vi "Initialise Waypoint GMap.vi"(7 "Aircraft ID":u8, 8 "error in (no error)":errorcluster, 11 "Main Map":refnum<k24>(container)) -> (0 "Error Out":errorcluster, 2 "Main Map Control Ref":refnum<k24>, 3 "Main map DLL Ref":refnum<k24>)   [LabVIEW 2014]
uses:
  C:/Robotic Systems/Products/AgFalcon/Software/Ground Station/Data/Mapping DLL/GMap.NET.WindowsForms.dll
  Data/Mapping DLL/GMap.NET.WindowsForms.dll
  C:/Robotic Systems/Products/AgFalcon/Software/Ground Station/Data/Mapping DLL/GMap.NET.Core.dll
  Data/Mapping DLL/GMap.NET.Core.dll
  Aircraft Information/Sub VI/Get Aircraft GPS.vi
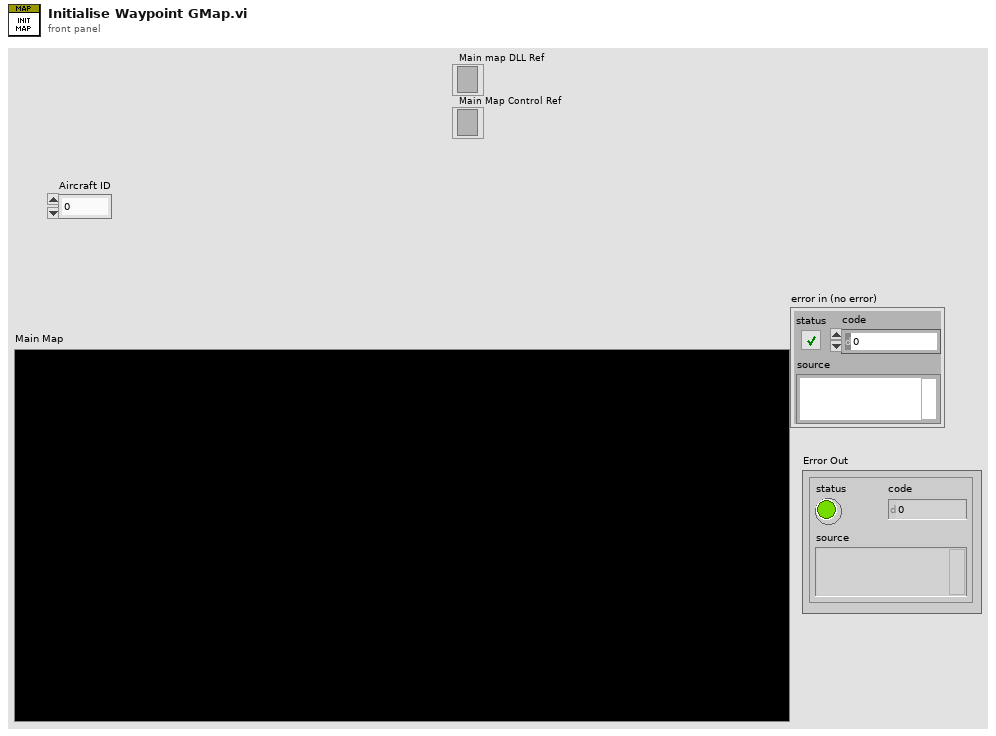
[diagram p1: front panel]
types:
  T1 = typedef "Aircraft GPS Data.ctl" = cluster{"Latitude (degrees)":dbl, "Longitude (degrees)":dbl, "Altitude (m)":dbl, "Fix Type":u8, "HDOP (cm)":u16, "VDOP (cm)":u16, "Ground Speed (m/s)":dbl, "Coarse Over Ground (degrees)":u16, "Number of Satellites":u8}
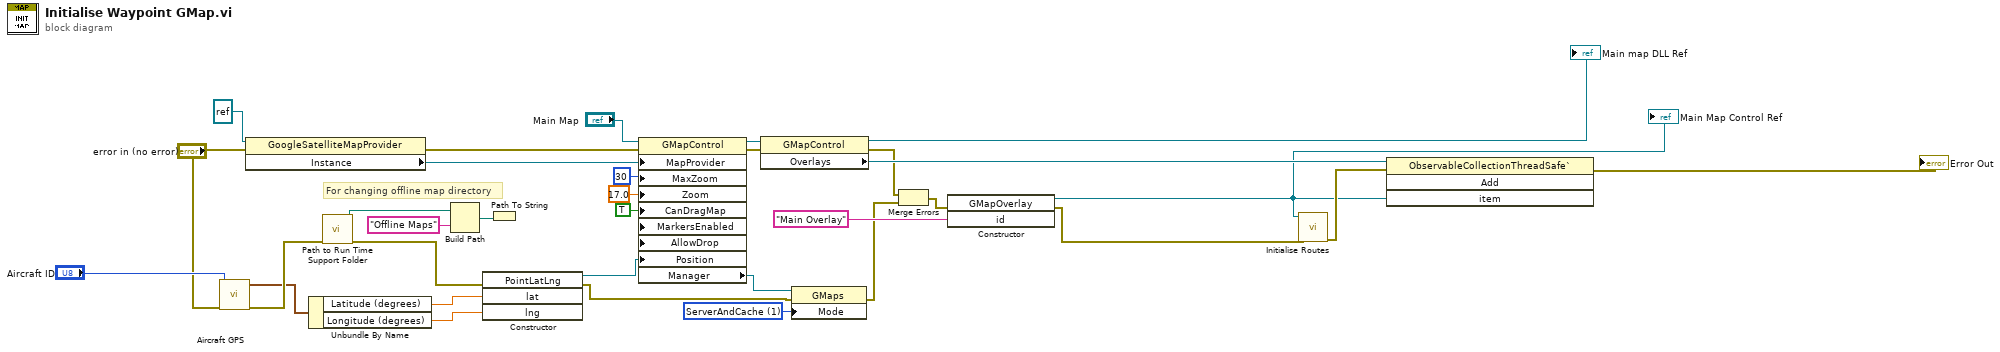
[diagram p0: block diagram]
diagram:
  w22 = 1 items=["ServerOnly", "ServerAndCache", "CacheOnly"] ("Mode")
  w27 = TRUE ("CanDragMap")
  # "For changing offline map directory"
  n1 = call-poly "Aircraft GPS.vi"("Error In"="error in (no error)", "Aircraft ID"="Aircraft ID") -> ("Error Out"=w4:errorcluster, "Aircraft GPS Data Out"=w3:T1)  [unwired: 8 in]
  n2 = property class="GoogleSatelliteMapProvider"(reference=refnum<k24> refnum (".NET Container Reference"), error in="error in (no error)") -> (error out=w33:errorcluster, "Instance"=w32:refnum<k24>)  [unwired: 1 out]
  n3 = Unbundle By Name(w3) -> ("Latitude (degrees)"=w2:dbl, "Longitude (degrees)"=w1:dbl)
  n4 = call "Path to Run Time Support Folder.vi"("Error In"=w4) -> ("Error Out"=w10:errorcluster, "Path To Run Time Support Folder"=w11:path)  [unwired: 9 in]
  n5 = Build Path(base path=w11, name or relative path="Offline Maps") -> (appended path=w12:path)
  n6 = constructor class="PointLatLng"(error in=w10, "lat"=w2, "lng"=w1) -> (reference out=w24:refnum<k24>, error out=w21:errorcluster)  [unwired: 2 in, 3 out]
  n7 = Path To String(path=w12) -> ()  [unwired: 1 out]
  n8 = property class="GMapControl"(reference="Main Map", error in=w33, "MapProvider"=w32, "MaxZoom"=30, "Zoom"=17.0, "CanDragMap"=w27, "MarkersEnabled"=w27, "AllowDrop"=w27, "Position"=w24) -> (reference out=w19:refnum<k24>, error out=w26:errorcluster, "Manager"=w23:refnum<k24>)
  n9 = property class="GMapControl"(reference=w19, error in=w26) -> (reference out=→"Main map DLL Ref":refnum<k24>, error out=w14:errorcluster, "Overlays"=w20:refnum<k24>)
  n10 = property class="GMaps"(reference=w23, error in=w21, "Mode"=w22) -> (error out=w13:errorcluster)  [unwired: 1 out]
  n11 = Merge Errors(w14, w13) -> (w15:errorcluster)
  n12 = constructor class="GMapOverlay"(error in=w15, "id"="Main Overlay") -> (reference out=w16:refnum<k24>, error out=w8:errorcluster)  [unwired: 2 in, 2 out]
  "Main Map Control Ref" <- w16
  n13 = call "Initialise Routes.vi"("error in (no error)"=w8, "Main Overlay"=w16) -> ("error out"=w18:errorcluster)  [unwired: 9 in]
  n14 = invoke class="ObservableCollectionThreadSafe`" method="Add"(reference=w20, error in=w18, "item"=w16) -> (error out=→"Error Out":errorcluster)  [unwired: 1 in, 3 out]
